vi "Stop Log.vi"(7 "VolatusAPI in":refnum<class "VolatusAPI.lvclass">, 8 "error in (no error)":errorcluster, 9 "Target (All)":string, 10 "Log Group (All)":T1, 11 "GroupLoggingControl in":refnum<class "GroupLoggingControl.lvclass">) -> (0 "error out":errorcluster, 3 "GroupLoggingControl out":refnum<class "GroupLoggingControl.lvclass">)   [LabVIEW 2020, in "VolatusGUIElements.lvlib" / "GroupLoggingControl.lvclass"]
uses:
  GroupLoggingControl.lvclass
  Log Group.ctl
  Log Group Status.ctl
  Command Info.ctl
  Volatus/VolatusAPI/VolatusAPI.lvclass
  messages/StopLog/Data.ctl
  GroupLoggingControl.lvclass/GroupLoggingControl.ctl
  messages/StopLog/Class/Msg.lvclass/Msg.ctl
  Volatus/VolatusAPI/VolatusAPI.lvclass/VolatusAPI.ctl
  messages/StopLog/Class/Msg.lvclass
  C:/dev/lv20CE/relink/lv-protoc/LV-Proto/Message/Message.lvclass
  lv-vecto/Vecto/TCPMessageService/Send Message.vi
  <vilib>/Utility/error.llb/Error Cluster From Error Code.vi
  lv-protoc/LV-Proto/Message/Message.lvclass
  messages/StopLog/StopLog.lvlib
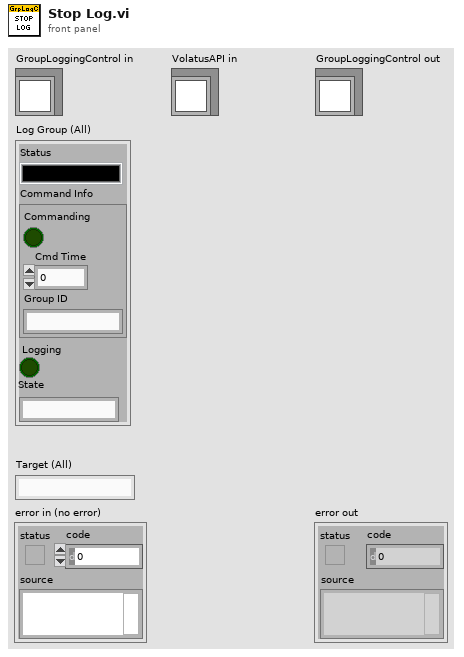
[diagram p1: front panel]
types:
  T1 = typedef "VolatusGUIElements.lvlib/GroupLoggingControl.lvclass/Log Group.ctl" = cluster{"Status":T2, "Command Info":T3, "Logging":bool, "State":string}
  T2 = typedef "VolatusGUIElements.lvlib/GroupLoggingControl.lvclass/Log Group Status.ctl" = cluster{"Group":string, "Group Color":u32, "Button":bool}
  T3 = typedef "VolatusGUIElements.lvlib/GroupLoggingControl.lvclass/Command Info.ctl" = cluster{"Commanding":bool, "Cmd Time":dbl, "Group ID":string}
  T4 = typedef "StopLog.lvlib/Data.ctl" = cluster{"reason":string, "groups":string[]}
  T5 = typedef "VolatusGUIElements.lvlib/GroupLoggingControl.lvclass/Target Info.ctl" = cluster{"Node":string, "Node Color":u32, "Groups":T1[]}
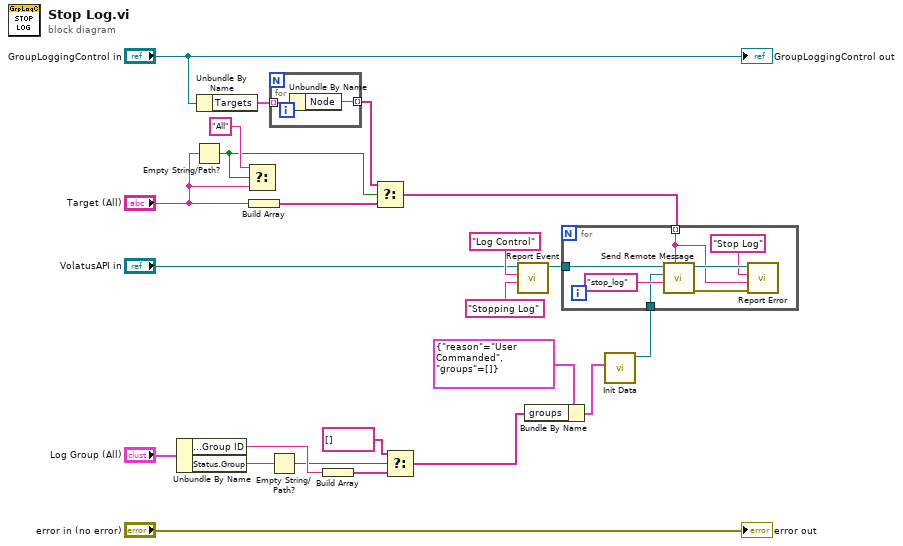
[diagram p0: block diagram]
diagram:
  n1 = Unbundle By Name("Log Group (All)") -> ("Command Info.Group ID"=w2:string, "Status.Group"=w7:string)
  n2 = Empty String/Path?(string/path="Target (All)") -> (empty?=w15:bool)
  n3 = Unbundle By Name("GroupLoggingControl in") -> ("Targets"=w16:T5[])
  n4 = Select(t="All", s=w15, f="Target (All)") -> ()  [unwired: 1 out]
  n5 = Build Array("Target (All)") -> (w13:string[])
  n6 = Empty String/Path?(string/path=w7) -> (empty?=w1:bool)
  n7 = for {
    tunnel: w16 -> [w25] mode=indexing
    tunnel: [w24] -> w14 mode=indexing
    n8 = Unbundle By Name(w25) -> ("Node"=w24:string)
  }
  n9 = Build Array(w2) -> (w6:string[])
  n10 = Select(t=w14, s=w15, f=w13) -> (s? t:f=w10:string[])
  n11 = Select(t=string[] [], s=w1, f=w6) -> (s? t:f=w3:string[])
  n12 = call "Report Event.vi"("Message"="Stopping Log" ("Context"), "Context"="Log Control", "VolatusAPI in"="VolatusAPI in") -> ("VolatusAPI out"=w21:refnum<class "VolatusAPI.lvclass">)  [unwired: 7 in, 1 out]
  n13 = Bundle By Name(cluster=T4 {"reason"="User Commanded", "groups"=[]} ("Data"), "groups"=w3) -> (w8:T4)
  n14 = call "Init Data.vi"("Data"=w8) -> ("Msg out"=w22:refnum<class "Msg.lvclass">)  [unwired: 10 in]
  n15 = for {
    tunnel: w21 -> [w32]
    tunnel: w10 -> [w27] mode=indexing
    tunnel: w22 -> [w26]
    n16 = call "Send Remote Message.vi"("Target Name"=w27, "Message Type"="stop_log", "Message"=w26, "VolatusAPI in"=w32) -> ("error out"=w28:errorcluster, "VolatusAPI out"=w31:refnum<class "VolatusAPI.lvclass">)  [unwired: 6 in]
    n17 = call "Report Error.vi"("error in (no error)"=w28, "Message"=w27, "Context"="Stop Log", "VolatusAPI in"=w31) -> ()  [unwired: 6 in, 2 out]
  }
  "error out" <- "error in (no error)"
  "GroupLoggingControl out" <- "GroupLoggingControl in"
